vi "Set_NavXAngle.vi"(9 "NavX Angle":dbl) -> ()   [LabVIEW 2016, in "DriveBase.lvclass"]
uses:
  DriveBase.lvclass
  DriveBase.lvclass/DriveBase.ctl
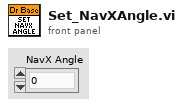
[diagram p1: front panel]
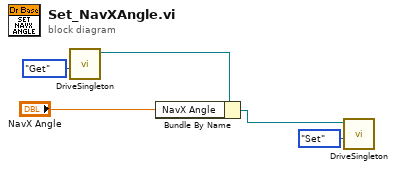
[diagram p0: block diagram]
diagram:
  n1 = call "DriveSingleton.vi"("Get/Set"=enum16{"Get", "Set"}."Get") -> ("DriveBase.lvclass 2"=w3:refnum<class "DriveBase.lvclass">)  [unwired: 9 in, 1 out]
  n2 = Bundle By Name(cluster=w3, "NavX Angle"="NavX Angle") -> (w1:refnum<class "DriveBase.lvclass">)
  n3 = call "DriveSingleton.vi"("Get/Set"=enum16{"Get", "Set"}."Set", "DriveBase.lvclass"=w1) -> ()  [unwired: 8 in, 2 out]
